vi "Experiment header-Bundle & save STATS section26_01_18.vi"(8 "error in (no error)":errorcluster, 11 "Logging queue element":T1 {"Ref Dwell time (us)" format="%#.6g"; "Frame Size" items=["100X100"=100, "128X128"=128, "200X200"=200, "256X256"=256, "512X512"=512, "1024x1024"=1024, "2048x2048"=2048]; "Dwell time (us)" format="%#.6g"}) -> (0 "error out":errorcluster)   [LabVIEW 2017]
uses:
  Typedefs/Logging queue element.ctl
  Typedefs/Imaging Protocols enum.ctl
  Typedefs/Frame Size.ctl
  Typedefs/Acquired points count.ctl
  Global Variables/General Globals.vi
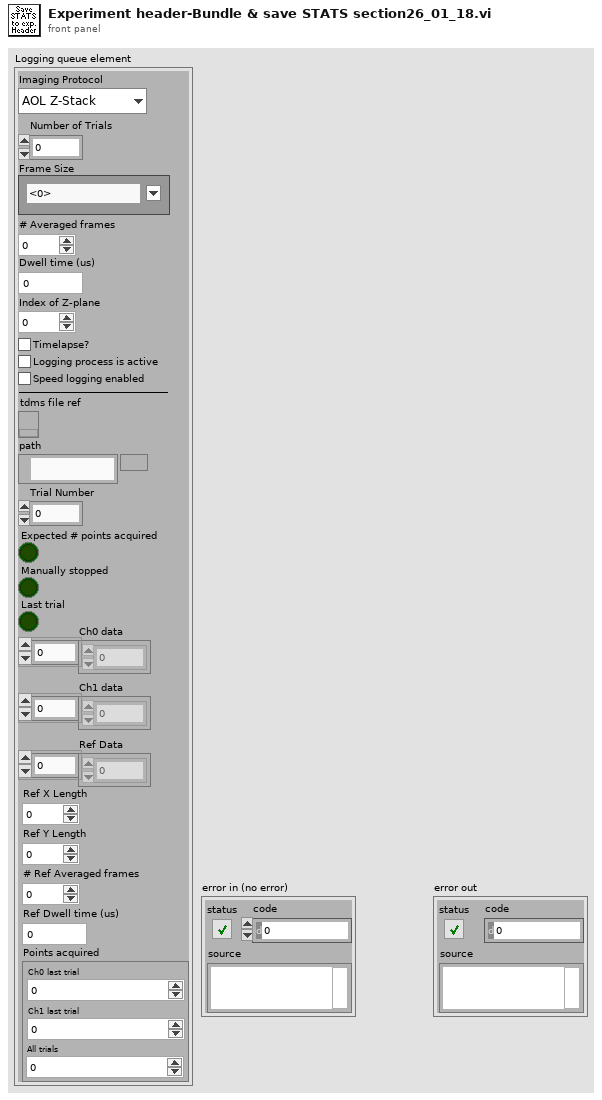
[diagram p1: front panel]
types:
  T1 = typedef "Logging queue element.ctl" = cluster{"Imaging Protocol":T2, "Number of Trials":u16, "Frame Size":T3, "# Averaged frames":u16, "Dwell time (us)":dbl, "Index of Z-plane":i32, "Timelapse?":bool, "Logging process is active":bool, "Speed logging enabled":bool, "tdms file ref":refnum<k34>, "path":path, "Trial Number":i32, "Expected # points acquired":bool, "Manually stopped":bool, "Ch0 data":u32[], "Ch1 data":u32[], "Ref Data":u32[], "Last trial":bool, "Ref Dwell time (us)":dbl, "# Ref Averaged frames":u16, "Ref X Length":u16, "Ref Y Length":u16, "Points acquired":T4}
  T2 = typedef "Imaging Protocols enum.ctl" = enum16{"AOL Z-Stack", "Motor Z Stack", "Functional Acquisition", "Single Plane Acquisition", "Volume Acquisition", "Live Imaging", "Live Plane Imaging", "Live Volume Imaging"}
  T3 = typedef "Frame Size.ctl" = u16
  T4 = typedef "Acquired points count.ctl" = cluster{"Ch0 last trial":u64, "Ch1 last trial":u64, "All trials":u64}
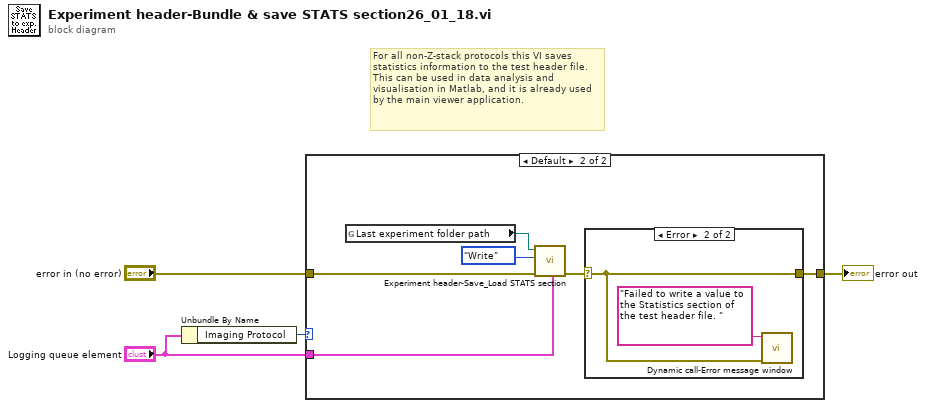
[diagram p0: block diagram]
diagram:
  # "For all non-Z-stack protocols this VI saves statistics information to the test header file.\nThis can be used in data analysis and visualisation in Matlab, and it is already used by the main viewer application."
  n1 = Unbundle By Name("Logging queue element") -> ("Imaging Protocol"=w2:T2)
  n2 = case shown="Default" w2 {
    tunnel: [w5 w6] -> w4
    tunnel: "error in (no error)" -> [w5 w11]
    tunnel: "Logging queue element" -> [_ w10]
    frame "AOL Z-Stack", "Motor Z Stack" {
    }
    frame Default {
      n3 = global read "General Globals.vi" "Last experiment folder path"() -> (w8:path)
      n4 = call "Experiment header-Save_Load STATS section.vi"("Logging queue element"=w10, "error in (no error)"=w11, "Function"=enum16{"Write", "Read"}."Write", "Experiment folder path"=w8) -> ("error out"=w7:errorcluster)  [unwired: 5 in, 2 out]
      n5 = case shown="Error" w7 {
        selector: w7 -> [w12 w13]
        tunnel: [w12 w13] -> w6
        frame No Error {
        }
        frame Error {
          n6 = call "Dynamic call-Error message window.vi"("error in (no error)"=w13, "Error Message"="Failed to write a value to the Statistics section of the test header file. ") -> ()  [unwired: 9 in, 1 out]
        }
      }
    }
  }
  "error out" <- w4
